vi "Write Q.vi"(8 "error in (no error)":errorcluster, 10 "Q":sgl, 11 "PAS Cell Data in":refnum<class "PAS Cell Data.lvclass">) -> (0 "error out":errorcluster, 3 "PAS Cell Data out":refnum<class "PAS Cell Data.lvclass">)   [LabVIEW 2017, in "PAS Library.lvlib" / "PAS Cell Data.lvclass"]
uses:
  PAS Cell Data.lvclass
  PAS Cell Data.lvclass/PAS Cell Data.ctl
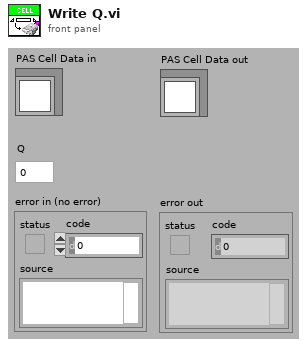
[diagram p1: front panel]
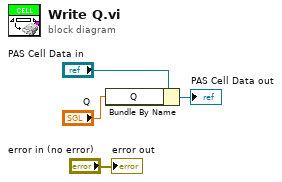
[diagram p0: block diagram]
diagram:
  n1 = Bundle By Name(cluster="PAS Cell Data in", "Q"="Q") -> (→"PAS Cell Data out":refnum<class "PAS Cell Data.lvclass">)
  "error out" <- "error in (no error)"
